vi "Event Handler.vi"(8 "error in (no error)":errorcluster, 10 "Stop Event Handler":refnum<user-event>, 11 "Calendar in":refnum<class "Calendar.lvclass">) -> (0 "error out":errorcluster)   [LabVIEW 2015, in "Calendar.lvclass"]
doc: "The <b>Event Handler VI</b> is a dynamic dispatch VI that should be overwritten if events are needed to create the enhanced QControl. \n\nBy inheriting from the main Control.lvclass the overwritten <b>Event Handler VI</b> will be launched asynchronously in the initialization of the QControl.\n<b> </b> <b> </b>\n©2016 Q Software Innovations, LLC (QSI)\nwritten by Quentin Alldredge\nproduced in LabVIEW 2015\n\nsupport@qsoftwareinnovations.com\nwww.qsoftwareinnovations.com\n\nAll rights reserved.\n\nRedistribution and use in source and binary forms, with or without modification, are permitted provided that the following conditions are met:\n\n * Redistributions of source code must retain the above copyright notice, this list of conditions and the following disclaimer.\n * Redistributions in binary form must reproduce the above copyright notice, this list of conditions and the following disclaimer in the documentation and/or other materials provided with the distribution.\n * Neither the name of Q Software Innovations, LLC. nor the names of its contributors may be used to endorse or promote products derived from this software without specific prior written permission.\n\nTHIS SOFTWARE IS PROVIDED BY THE COPYRIGHT HOLDERS AND CONTRIBUTORS \"AS IS\" AND ANY EXPRESS OR IMPLIED WARRANTIES, INCLUDING, BUT NOT LIMITED TO, THE IMPLIED WARRANTIES OF MERCHANTABILITY AND FITNESS FOR A PARTICULAR PURPOSE ARE DISCLAIMED. IN NO EVENT SHALL THE COPYRIGHT OWNER OR CONTRIBUTORS BE LIABLE FOR ANY DIRECT, INDIRECT, INCIDENTAL, SPECIAL, EXEMPLARY, OR CONSEQUENTIAL DAMAGES (INCLUDING, BUT NOT LIMITED TO, PROCUREMENT OF SUBSTITUTE GOODS OR SERVICES; LOSS OF USE, DATA, OR PROFITS; OR BUSINESS INTERRUPTION) HOWEVER CAUSED AND ON ANY THEORY OF LIABILITY, WHETHER IN CONTRACT, STRICT LIABILITY, OR TORT (INCLUDING NEGLIGENCE OR OTHERWISE) ARISING IN ANY WAY OUT OF THE USE OF THIS SOFTWARE, EVEN IF ADVISED OF THE POSSIBILITY OF SUCH DAMAGE."
uses:
  Calendar.lvclass
  <vilib>/Utility/miscctls.llb/LVPoint32TypeDef.ctl
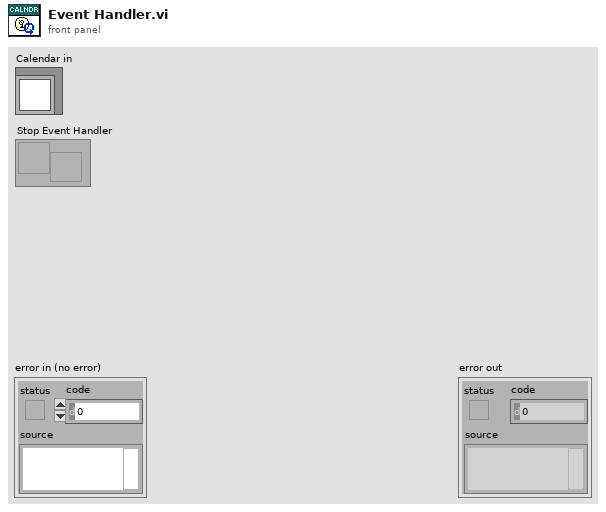
[diagram p1: front panel]
types:
  T1 = typedef "LVPoint32TypeDef.ctl" = cluster{"Horizontal":i32, "Vertical":i32}
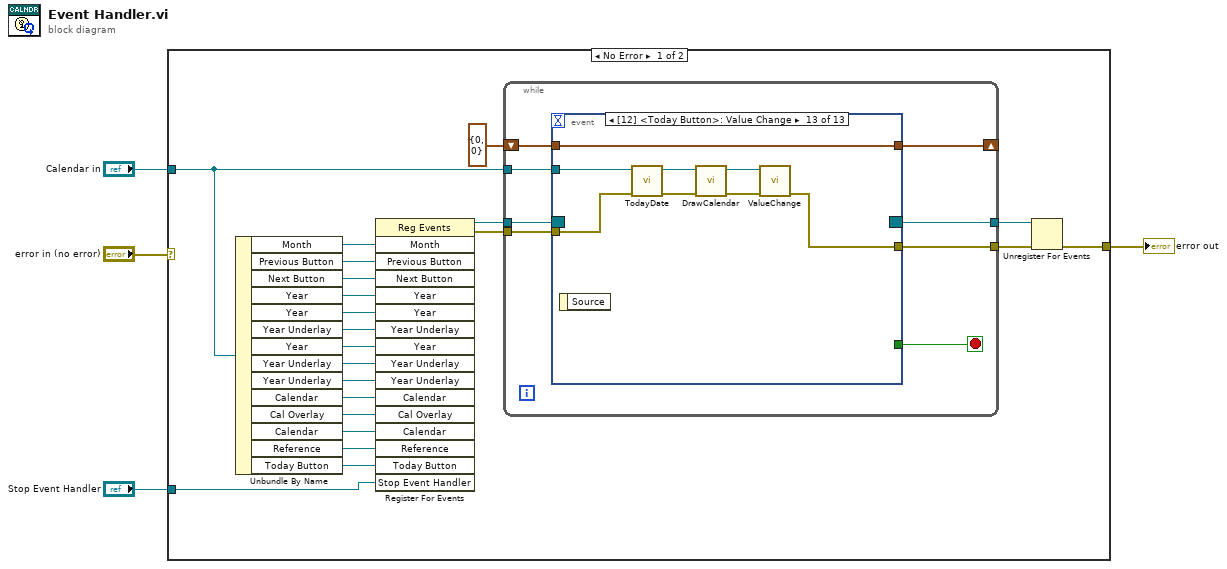
[diagram p0: block diagram]
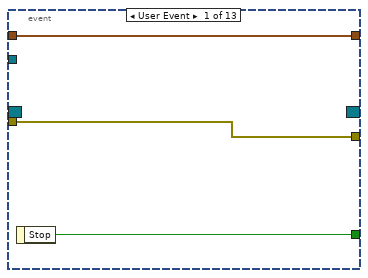
[diagram p2: hidden frame]
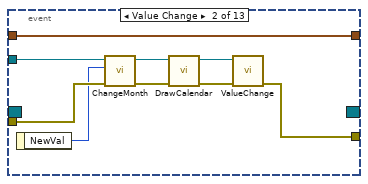
[diagram p3: hidden frame]
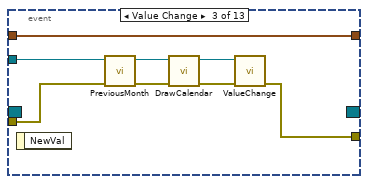
[diagram p4: hidden frame]
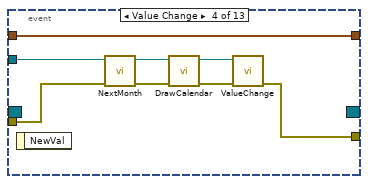
[diagram p5: hidden frame]
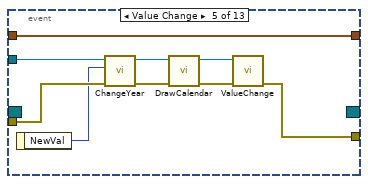
[diagram p6: hidden frame]
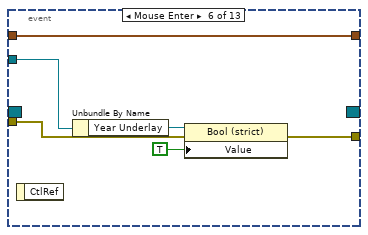
[diagram p7: hidden frame]
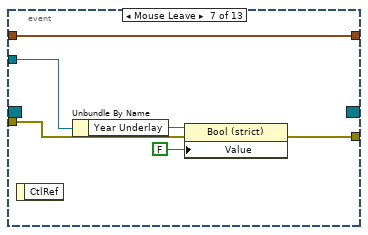
[diagram p8: hidden frame]
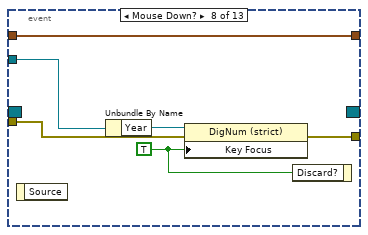
[diagram p9: hidden frame]
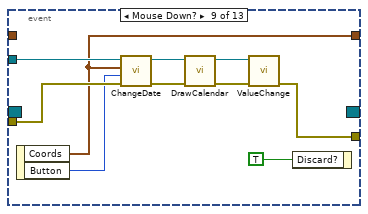
[diagram p10: hidden frame]
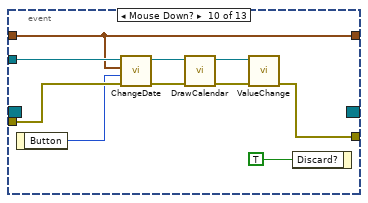
[diagram p11: hidden frame]
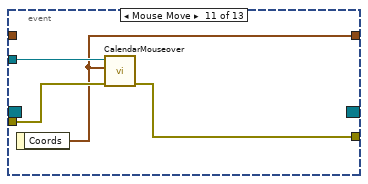
[diagram p12: hidden frame]
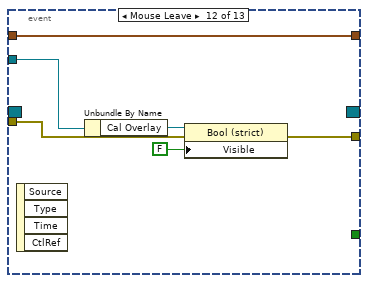
[diagram p13: hidden frame]
diagram:
  n1 = case shown="No Error" "error in (no error)" {
    selector: "error in (no error)" -> [_ w128]
    tunnel: [w23 w128] -> w3
    tunnel: "Calendar in" -> [w21 _]
    tunnel: "Stop Event Handler" -> [w19 _]
    frame No Error {
      n2 = Unbundle By Name(w21) -> ("Month"=w20:refnum<vi>, "Previous Button"=w18:refnum<vi>, "Next Button"=w17:refnum<vi>, "Year"=w16:refnum<vi>, "Year"=w15:refnum<vi>, "Year Underlay"=w14:refnum<vi>, "Year"=w13:refnum<vi>, "Year Underlay"=w12:refnum<vi>, "Year Underlay"=w11:refnum<vi>, "Calendar"=w10:refnum<vi>, "Cal Overlay"=w8:refnum<vi>, "Calendar"=w7:refnum<vi>, "Reference"=w6:refnum<vi>, "Today Button"=w5:refnum<vi>)
      n3 = register-events(w20, w18, w17, w16, w15, w14, w13, w12, w11, w10, w8, w7, w6, w5, w19) -> (reference out=w26:refnum<event-registration>, error out=w25:errorcluster)  [unwired: 2 in]
      n4 = while {
        tunnel: w26 -> [w34]
        tunnel: w25 -> [w32]
        tunnel: [w31] -> w24
        tunnel: [w27] -> w22
        tunnel: w21 -> [w33]
        shift-right: [w29] -> _
        shift-left: T1 {"Horizontal"=0, "Vertical"=0} ("Coords") -> [w28]
        stop <- w30 stop-if-true
        n5 = event shown="[12] <Today Button>: Value Change" {
          selector: w34 -> [_ _ _ _ _ _ _ _ _ _ _ _ _]
          dyn-events: [_ _ _ _ _ _ _ _ _ _ _ _ _] -> w27
          timeout: _ -> [_ _ _ _ _ _ _ _ _ _ _ _ _]
          tunnel: w33 -> [_ w46 w54 w62 w71 w72 w78 w84 w99 w109 w113 w114 w127]
          tunnel: w32 -> [w37 w45 w53 w61 w70 w74 w80 w87 w98 w108 w112 w116 w126]
          tunnel: [w37 w38 w47 w55 w63 w75 w81 w88 w91 w101 w110 w117 w120] -> w31
          tunnel: [w36 _ _ _ _ _ _ _ _ _ _ _ _] -> w30
          tunnel: [w35 w43 w52 w60 w68 w73 w79 w85 w96 w106 w111 w115 w125] -> w29
          tunnel: w28 -> [w35 w43 w52 w60 w68 w73 w79 w85 _ w106 _ w115 w125]
          event User Event {
            n6 = event-data() -> ("Stop"=w36:bool)  [unwired: 1 in]
          }
          event Value Change {
            n7 = event-data() -> ("NewVal"=w44:u16)  [unwired: 1 in]
            n8 = call "ChangeMonth.vi"("error in (no error)"=w45, "Month"=w44, "Calendar in"=w46) -> ("error out"=w41:errorcluster, "Calendar (dup)"=w42:refnum<class "Calendar.lvclass">)  [unwired: 7 in]
            n9 = call "DrawCalendar.vi"("error in (no error)"=w41, "Calendar in"=w42) -> ("error out"=w39:errorcluster, "Calendar out"=w40:refnum<class "Calendar.lvclass">)  [unwired: 8 in]
            n10 = call "ValueChange.vi"("error in (no error)"=w39, "Calendar in"=w40) -> ("error out"=w38:errorcluster)  [unwired: 8 in, 1 out]
          }
          event Value Change {
            n11 = event-data() -> ()  [unwired: 1 in, 1 out]
            n12 = call "PreviousMonth.vi"("error in (no error)"=w53, "Calendar in"=w54) -> ("error out"=w50:errorcluster, "Calendar (dup)"=w51:refnum<class "Calendar.lvclass">)  [unwired: 8 in]
            n13 = call "DrawCalendar.vi"("error in (no error)"=w50, "Calendar in"=w51) -> ("error out"=w48:errorcluster, "Calendar out"=w49:refnum<class "Calendar.lvclass">)  [unwired: 8 in]
            n14 = call "ValueChange.vi"("error in (no error)"=w48, "Calendar in"=w49) -> ("error out"=w47:errorcluster)  [unwired: 8 in, 1 out]
          }
          event Value Change {
            n15 = event-data() -> ()  [unwired: 1 in, 1 out]
            n16 = call "NextMonth.vi"("error in (no error)"=w61, "Calendar in"=w62) -> ("error out"=w58:errorcluster, "Calendar (dup)"=w59:refnum<class "Calendar.lvclass">)  [unwired: 8 in]
            n17 = call "DrawCalendar.vi"("error in (no error)"=w58, "Calendar in"=w59) -> ("error out"=w56:errorcluster, "Calendar out"=w57:refnum<class "Calendar.lvclass">)  [unwired: 8 in]
            n18 = call "ValueChange.vi"("error in (no error)"=w56, "Calendar in"=w57) -> ("error out"=w55:errorcluster)  [unwired: 8 in, 1 out]
          }
          event Value Change {
            n19 = event-data() -> ("NewVal"=w69:i32)  [unwired: 1 in]
            n20 = call "ChangeYear.vi"("error in (no error)"=w70, "Year"=w69, "Calendar in"=w71) -> ("error out"=w66:errorcluster, "Calendar (dup)"=w67:refnum<class "Calendar.lvclass">)  [unwired: 7 in]
            n21 = call "DrawCalendar.vi"("error in (no error)"=w66, "Calendar in"=w67) -> ("error out"=w64:errorcluster, "Calendar out"=w65:refnum<class "Calendar.lvclass">)  [unwired: 8 in]
            n22 = call "ValueChange.vi"("error in (no error)"=w64, "Calendar in"=w65) -> ("error out"=w63:errorcluster)  [unwired: 8 in, 1 out]
          }
          event Mouse Enter {
            n23 = event-data() -> ()  [unwired: 1 in, 1 out]
            n24 = Unbundle By Name(w72) -> ("Year Underlay"=w77:refnum<vi>)
            n25 = property class="Bool (strict)"(reference=w77, error in=w74, "Value"=TRUE ("Visible")) -> (error out=w75:errorcluster)  [unwired: 1 out]
          }
          event Mouse Leave {
            n26 = event-data() -> ()  [unwired: 1 in, 1 out]
            n27 = Unbundle By Name(w78) -> ("Year Underlay"=w83:refnum<vi>)
            n28 = property class="Bool (strict)"(reference=w83, error in=w80, "Value"=FALSE ("Visible")) -> (error out=w81:errorcluster)  [unwired: 1 out]
          }
          event Mouse Down? {
            w86 = TRUE ("Visible")
            n29 = event-data() -> ()  [unwired: 1 in, 1 out]
            n30 = Unbundle By Name(w84) -> ("Year"=w89:refnum<vi>)
            n31 = property class="DigNum (strict)"(reference=w89, error in=w87, "Key Focus"=w86) -> (error out=w88:errorcluster)  [unwired: 1 out]
            n32 = event-data("Discard?"=w86) -> ()  [unwired: 1 in, 1 out]
          }
          event Mouse Down? {
            n33 = event-data() -> ("Coords"=w96:T1, "Button"=w97:u16)  [unwired: 1 in]
            n34 = call "ChangeDate.vi"("error in (no error)"=w98, "Button"=w97, "Coords"=w96, "Calendar in"=w99) -> ("error out"=w94:errorcluster, "Calendar (dup)"=w95:refnum<class "Calendar.lvclass">)  [unwired: 6 in]
            n35 = call "DrawCalendar.vi"("error in (no error)"=w94, "Calendar in"=w95) -> ("error out"=w92:errorcluster, "Calendar out"=w93:refnum<class "Calendar.lvclass">)  [unwired: 8 in]
            n36 = call "ValueChange.vi"("error in (no error)"=w92, "Calendar in"=w93) -> ("error out"=w91:errorcluster)  [unwired: 8 in, 1 out]
            n37 = event-data("Discard?"=TRUE) -> ()  [unwired: 1 in, 1 out]
          }
          event Mouse Down? {
            n38 = event-data() -> ("Button"=w107:u16)  [unwired: 1 in]
            n39 = call "ChangeDate.vi"("error in (no error)"=w108, "Button"=w107, "Coords"=w106, "Calendar in"=w109) -> ("error out"=w104:errorcluster, "Calendar (dup)"=w105:refnum<class "Calendar.lvclass">)  [unwired: 6 in]
            n40 = call "DrawCalendar.vi"("error in (no error)"=w104, "Calendar in"=w105) -> ("error out"=w102:errorcluster, "Calendar out"=w103:refnum<class "Calendar.lvclass">)  [unwired: 8 in]
            n41 = call "ValueChange.vi"("error in (no error)"=w102, "Calendar in"=w103) -> ("error out"=w101:errorcluster)  [unwired: 8 in, 1 out]
            n42 = event-data("Discard?"=TRUE) -> ()  [unwired: 1 in, 1 out]
          }
          event Mouse Move {
            n43 = event-data() -> ("Coords"=w111:T1)  [unwired: 1 in]
            n44 = call "CalendarMouseover.vi"("error in (no error)"=w112, "Coords"=w111, "Calendar in"=w113) -> ("error out"=w110:errorcluster)  [unwired: 7 in, 1 out]
          }
          event Mouse Leave {
            n45 = event-data() -> ()  [unwired: 1 in, 4 out]
            n46 = Unbundle By Name(w114) -> ("Cal Overlay"=w119:refnum<vi>)
            n47 = property class="Bool (strict)"(reference=w119, error in=w116, "Visible"=FALSE) -> (error out=w117:errorcluster)  [unwired: 1 out]
          }
          event Value Change {
            n48 = event-data() -> ()  [unwired: 1 in, 1 out]
            n49 = call "TodayDate.vi"("error in (no error)"=w126, "Calendar in"=w127) -> ("error out"=w123:errorcluster, "Calendar (dup)"=w124:refnum<class "Calendar.lvclass">)  [unwired: 8 in]
            n50 = call "DrawCalendar.vi"("error in (no error)"=w123, "Calendar in"=w124) -> ("error out"=w121:errorcluster, "Calendar out"=w122:refnum<class "Calendar.lvclass">)  [unwired: 8 in]
            n51 = call "ValueChange.vi"("error in (no error)"=w121, "Calendar in"=w122) -> ("error out"=w120:errorcluster)  [unwired: 8 in, 1 out]
          }
        }
      }
      n52 = Unregister For Events(event registration refnum=w22, error in=w24) -> (error out=w23:errorcluster)
    }
    frame Error {
    }
  }
  "error out" <- w3
